vi "terminate.vi"(8 "error in (no error)":errorcluster, 11 "SignalReaderCN091129DAQmx in":refnum<class "SignalReaderCN091129DAQmx.lvclass">) -> (0 "error out":errorcluster, 3 "SignalReaderCN091129DAQmx out":refnum<class "SignalReaderCN091129DAQmx.lvclass">)   [LabVIEW 2010, in "SignalReaderCN091129DAQmx.lvclass"]
doc: "The dynamic dispatch version of this VI terminates the plug-in object by releasing all of its resources."
uses:
  SignalReaderCN091129DAQmx.lvclass
  SignalReaderCN091129DAQmx.lvclass/SignalReaderCN091129DAQmx.ctl
  GenericSignalReader/GenericSignalReader/GenericSignalReader.lvclass
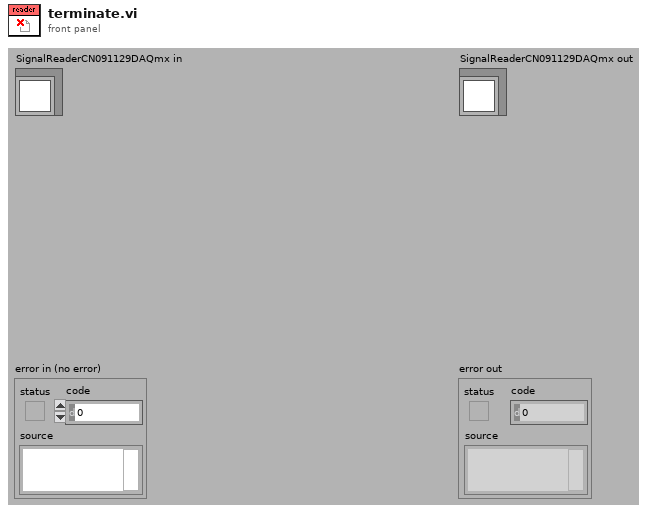
[diagram p1: front panel]
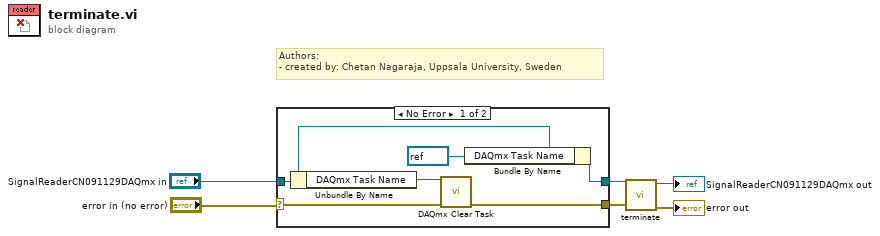
[diagram p0: block diagram]
diagram:
  # "Authors: \n- created by: Chetan Nagaraja, Uppsala University, Sweden"
  n1 = case shown="No Error" "error in (no error)" {
    selector: "error in (no error)" -> [w12 w14]
    tunnel: [w11 w14] -> w6
    tunnel: "SignalReaderCN091129DAQmx in" -> [w8 w13]
    tunnel: [w7 w13] -> w1
    frame No Error {
      n2 = Unbundle By Name(w8) -> ("DAQmx Task Name"=w10:refnum<k21>)
      n3 = call <vilib>:"DAQmx Clear Task.vi"("task in"=w10, "error in"=w12) -> ("error out"=w11:errorcluster)  [unwired: 13 in]
      n4 = Bundle By Name(cluster=w8, "DAQmx Task Name"=refnum<k21> refnum) -> (w7:refnum<class "SignalReaderCN091129DAQmx.lvclass">)
    }
    frame Error {
    }
  }
  n5 = call-parent "terminate.vi"("error in (no error)"=w6, "GenericPlugin in"=w1) -> ("error out"=→"error out":errorcluster, "GenericPlugin out"=→"SignalReaderCN091129DAQmx out":refnum<class "SignalReaderCN091129DAQmx.lvclass">)  [unwired: 8 in]
